vi "Target State Change Event Callback.vi"(4 "Target State User Event":refnum<user-event>, 5 "Event Data":cluster{"sender":refnum<k24>, "e":refnum<k24>}, 6 "Control Ref":refnum<k24>, 7 "Event Common Data":T1) -> ()   [LabVIEW 2020, in "NI_VS Workspace ExecutionAPI.lvlib"]
uses:
  <vilib>/NI VeriStand/Execution/Workspace/NI_VS Workspace ExecutionAPI.lvlib
  NationalInstruments.VeriStand.ClientAPI
  <vilib>/NI VeriStand/Execution/Workspace/Target State Info.ctl
  <vilib>/NI VeriStand/Execution/Workspace/Target State.ctl
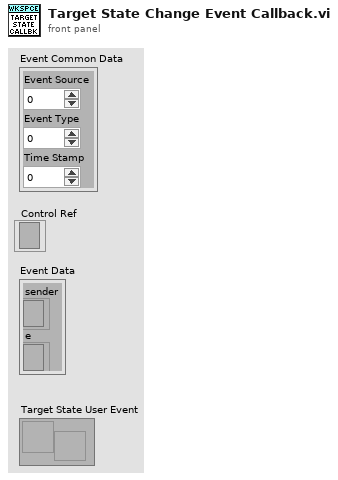
[diagram p1: front panel]
types:
  T1 = cluster{"Event Source":i32, "Event Type":u32, "Time Stamp":u32}
  T2 = typedef "NI_VS Workspace ExecutionAPI.lvlib/Target State Info.ctl" = cluster{"Target":string, "State":T3}
  T3 = typedef "NI_VS Workspace ExecutionAPI.lvlib/Target State.ctl" = enum16{"Disconnected", "Running", "Idle", "Disabled", "Connecting"}
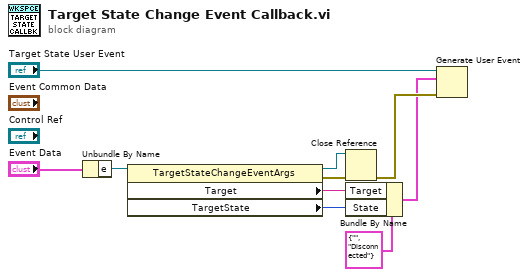
[diagram p0: block diagram]
diagram:
  n1 = Unbundle By Name("Event Data") -> ("e"=w8:refnum<k24>)
  n2 = property class="TargetStateChangeEventArgs"(reference=w8) -> (reference out=w7:refnum<k24>, error out=w6:errorcluster, "Target"=w2:string, "TargetState"=w1:i32)  [unwired: 1 in]
  n3 = Close Reference(reference=w7, error in (no error)=w6) -> (error out=w10:errorcluster)
  n4 = Bundle By Name(cluster=T2 {"Target"="", "State"=enum."Disconnected"} ("event data"), "Target"=w2, "State"=w1) -> (w3:T2)
  n5 = Generate User Event(user event="Target State User Event", event data cluster=w3, error in=w10) -> ()  [unwired: 1 in, 2 out]
